vi "Read Speed.vi"(8 "error in (no error)":errorcluster, 11 "Tool Object in":refnum<class "Tool Object.lvclass">) -> (0 "error out":errorcluster, 2 "Speed":dbl[](array[numeric]), 3 "Tool Object out":refnum<class "Tool Object.lvclass">)   [LabVIEW 2019, in "Tool Object.lvclass"]
uses:
  Tool Object.lvclass
  Tool Object.lvclass/Tool Object.ctl
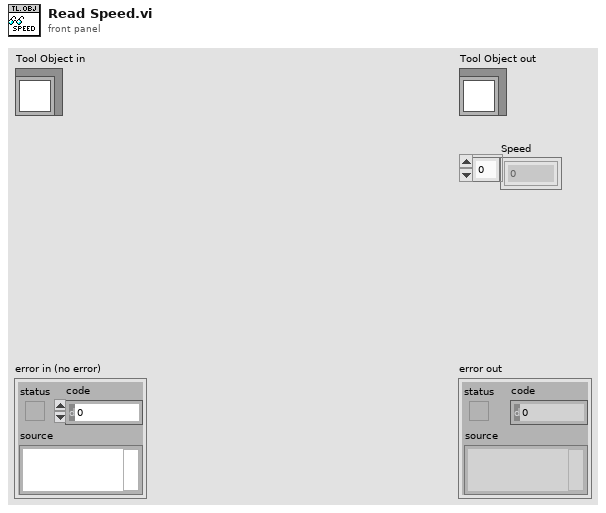
[diagram p1: front panel]
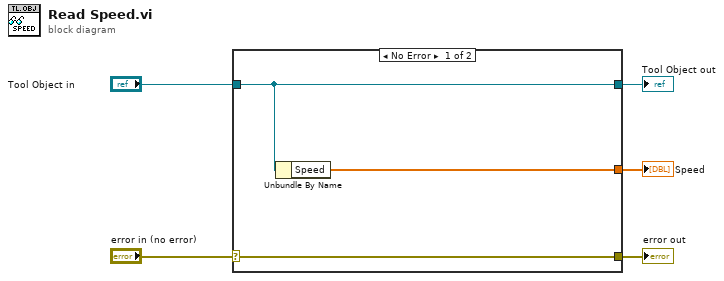
[diagram p0: block diagram]
diagram:
  n1 = case shown="No Error" "error in (no error)" {
    selector: "error in (no error)" -> [w8 w9]
    tunnel: [w8 w9] -> w4
    tunnel: [w7 w10] -> w2
    tunnel: "Tool Object in" -> [w7 w10]
    tunnel: [w6 _] -> w1
    frame No Error {
      n2 = Unbundle By Name(w7) -> ("Speed"=w6:dbl[])
    }
    frame Error {
    }
  }
  "error out" <- w4
  "Tool Object out" <- w2
  "Speed" <- w1
